vi "Main.vi"() -> ()   [LabVIEW 2021, in "Game of Life.lvlib"]
doc: "This template is for the Queued Message Handler design pattern.\n\nThe Event Handling Loop generates messages based on user interface actions.\n\nThe Message Handling Loop processes messages generated by the Event Handling Loop, or by other messages. The messages are string values, so new messages can be added easily to the Message Cases case structure in the Message Handling Loop. Each message cluster can also provide an optional value for Message Data, which is a variant that can be converted to whatever message-specific data is required."
uses:
  Game of Life.lvlib
  <vilib>/Plug-In SDKs/InstrumentStudio SDK/InstrumentStudioPluginSDK.lvlibp/Plugin Events Enum.ctl
  controls/Data.ctl
  controls/Configuration.ctl
  controls/Game of Life.ctl
  a2cd5499-92a9-455c-b0f9-1db12e3f6067.vi
  aef85ed4-6d5b-4a62-8cd4-232f16e6ae51.vi
  a2cd5499-92a9-455c-b0f9-1db12e3f6067.vi/6651a77e-856e-4bcd-af5a-c0c13b264cc1.vi
  aef85ed4-6d5b-4a62-8cd4-232f16e6ae51.vi/331b549c-fcf8-43d9-8a1e-5b3c0091a99c.vi
  <vilib>/JDP Science/JSONtext/JSON text to Variant.vi
  <vilib>/Utility/error.llb/Error Cluster From Error Code.vi
  <vilib>/JDP Science/JSONtext/Variant to JSON Text.vi
  <vilib>/JDP Science/JSONtext/LVClass Serializer/JSONtext LVClass Serializer.lvclass
  <vilib>/ErrorRing/Error Ring.xnode
  <vilib>/Plug-In SDKs/InstrumentStudio SDK/InstrumentStudioPluginSDK.lvlibp/Plugin Session.lvclass
  <vilib>/Plug-In SDKs/InstrumentStudio SDK/InstrumentStudioPluginSDK.lvlibp
panel:
  in  "Tab Control":enum32{"Game Panel", "Events"}(tab)
  in  "Start":bool
  out "game of life":T1(graph)
  out "generation":u32 caption="Generation"
  in  "update interval":u32=250 caption="Update interval (msec)" min=50
  in  "height":u32=100 caption="Board height" min=10
  in  "width":u32=100 caption="Board width" min=10
  in  "Log Events?":bool
  out "Event Record":i32(listbox)
  in  "Session Id":u64
  # "Enable Logging: Check this box to generate a log file and save the event record."
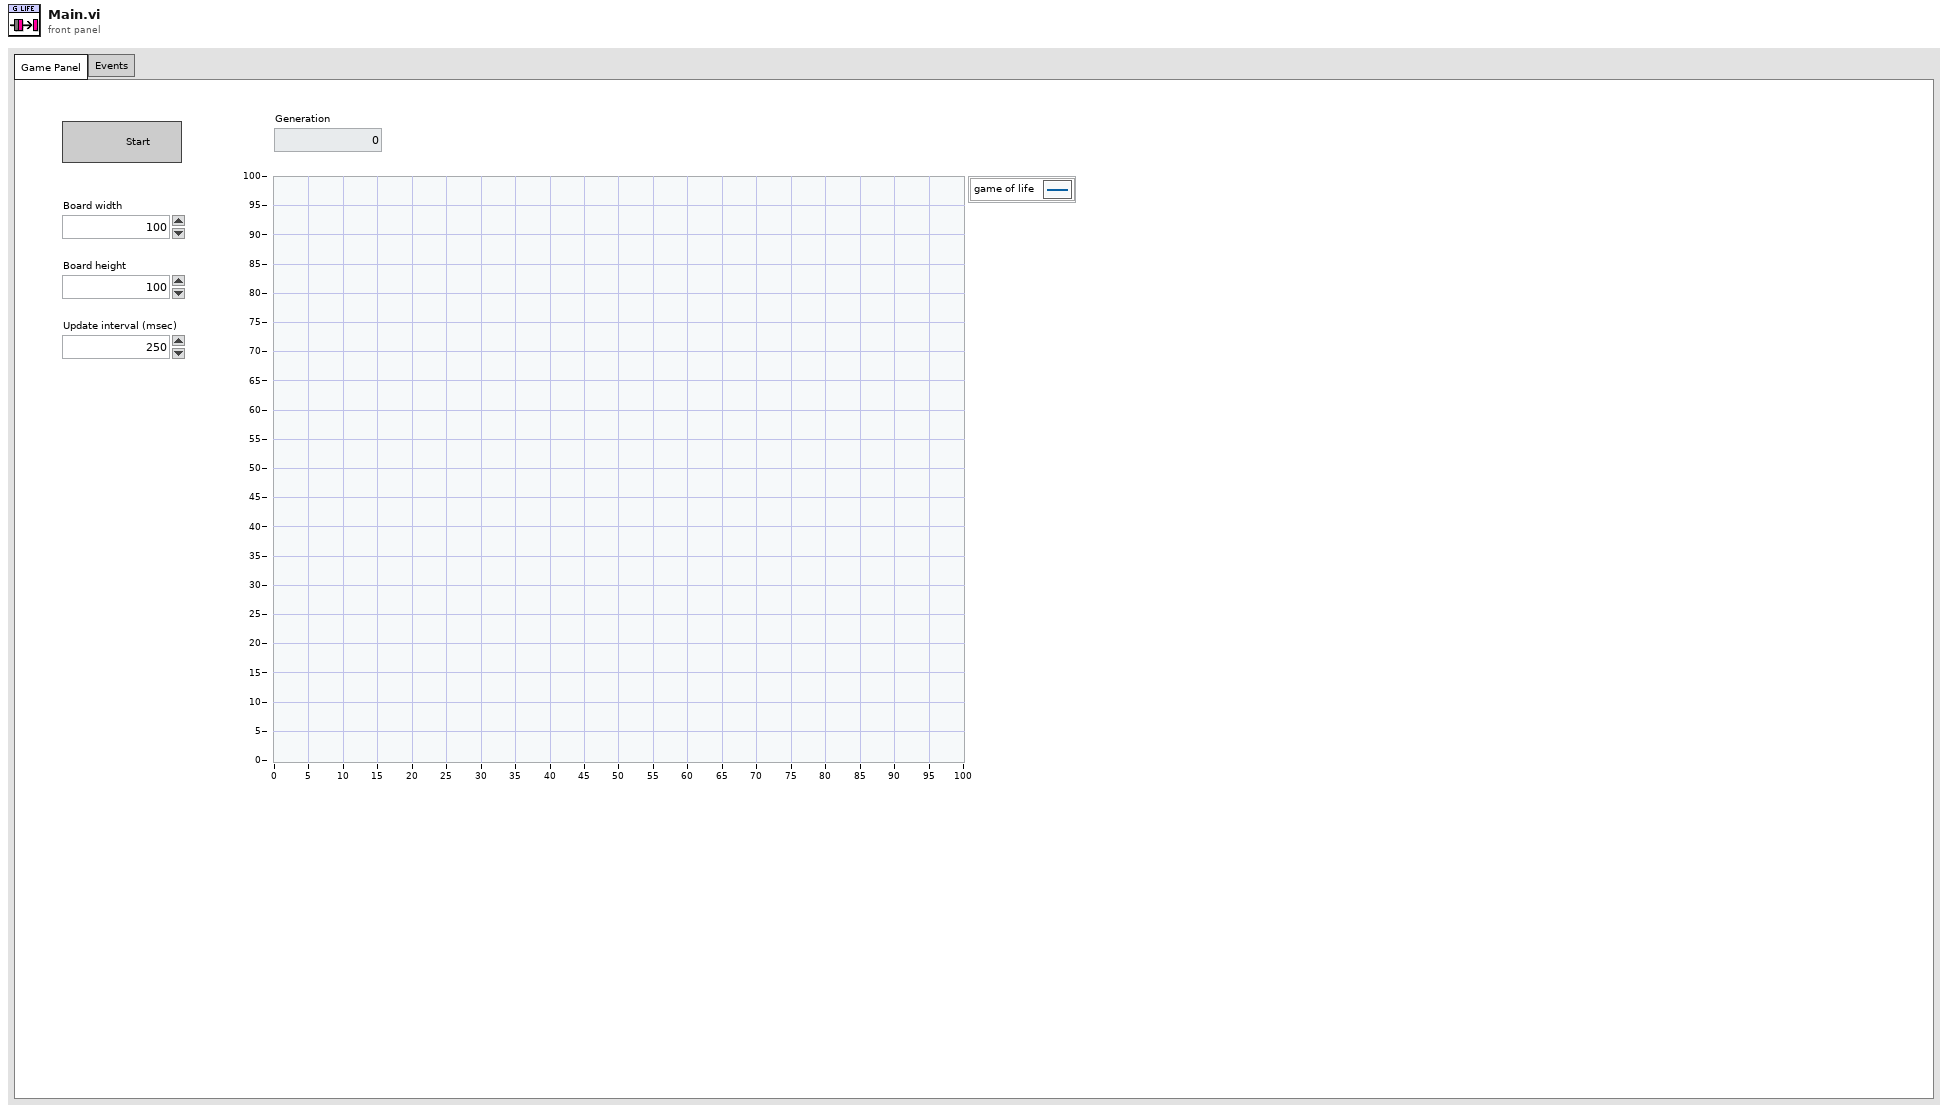
[diagram p1: front panel]
types:
  T1 = typedef "Game of Life.lvlib/Game of Life.ctl" = cluster{"x_data":dbl[], "y_data":dbl[]}
  T2 = typedef "Game of Life.lvlib/Data.ctl" = cluster{"Configuration":T3, "Generation":u32, "Run?":bool, "Cells":bool[][], "Log Events?":bool}
  T3 = typedef "Game of Life.lvlib/Configuration.ctl" = cluster{"Height":u32, "Width":u32, "Update Interval":u32}
  T4 = typedef "InstrumentStudioPluginSDK.lvlibp/Plugin Events Enum.ctl" = enum16{"Shutdown", "Project Saved", "Stop All Outputs"}
  T5 = typedef "InstrumentStudioPluginSDK.lvlibp/Event Registration Refnum.ctl" = refnum<event-registration>
  T6 = typedef "Game of Life.lvlib/All Message Queues.ctl" = cluster{"UI":refnum<queue>}
  T7 = cluster{"Event Refnum":T5, "Event Registration Refnum":refnum<event-registration>}
  T8 = enum8{"Enabled", "Disabled", "Disabled and Grayed Out"}
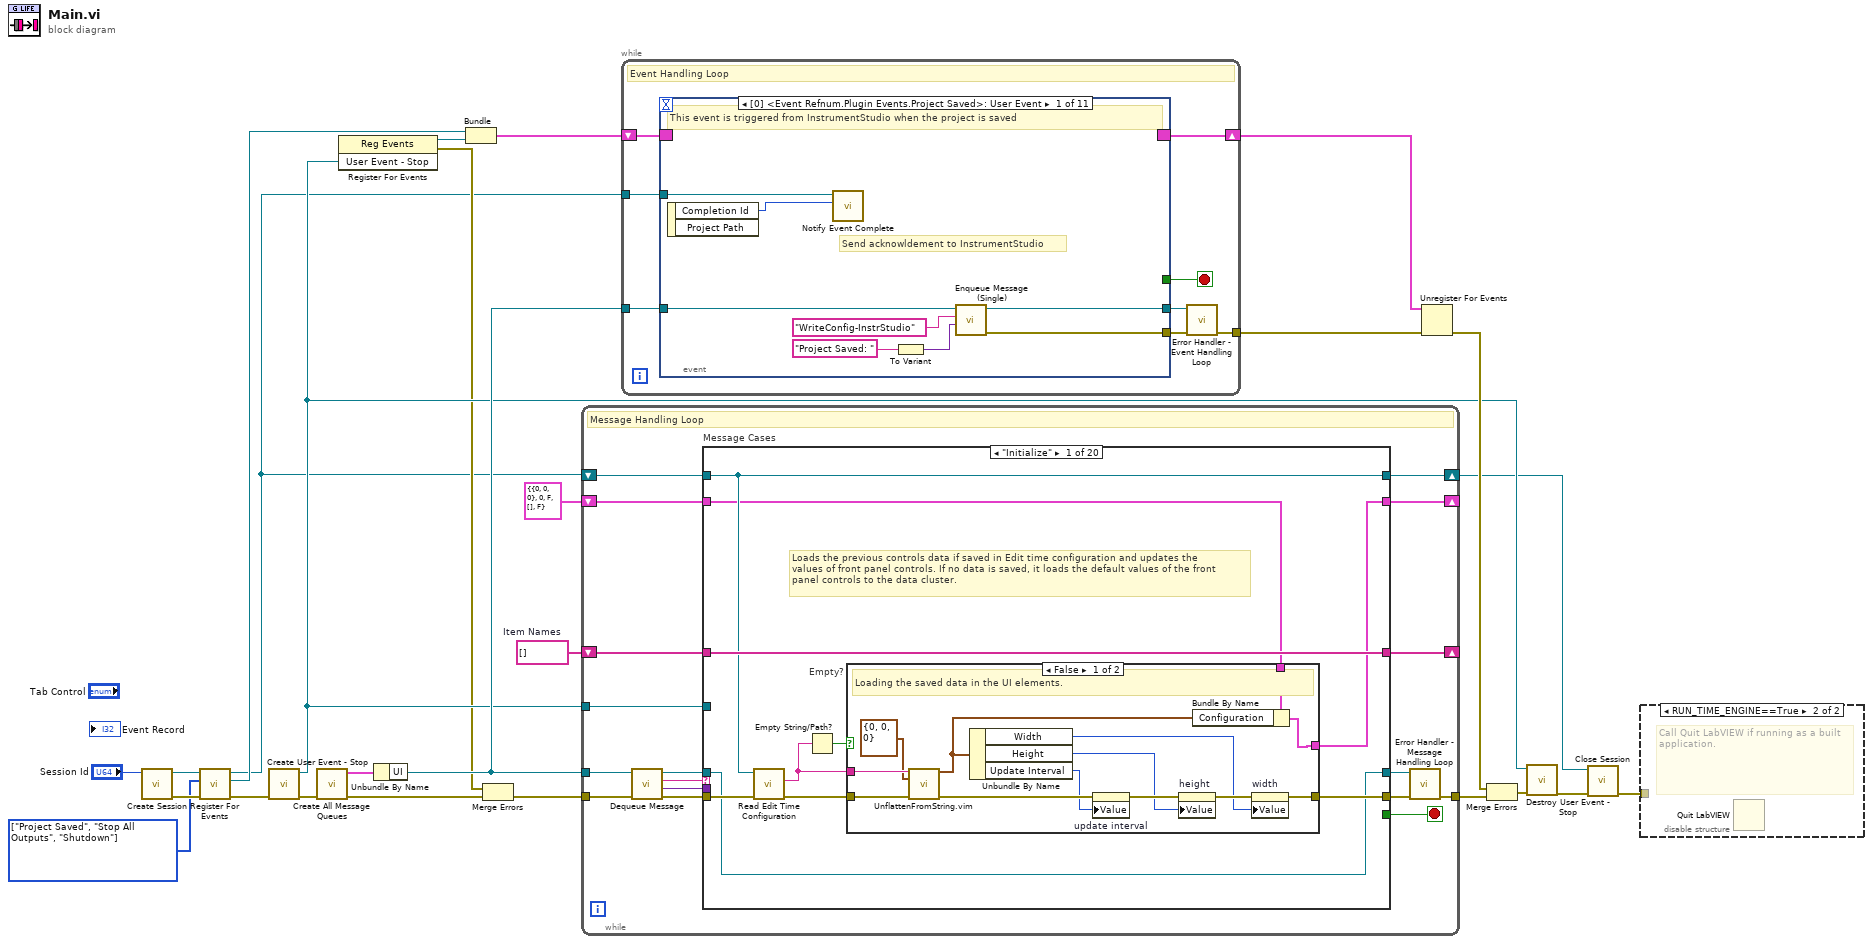
[diagram p0: block diagram]
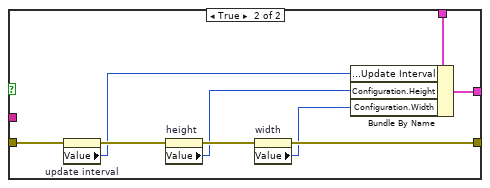
[diagram p3: hidden frame]
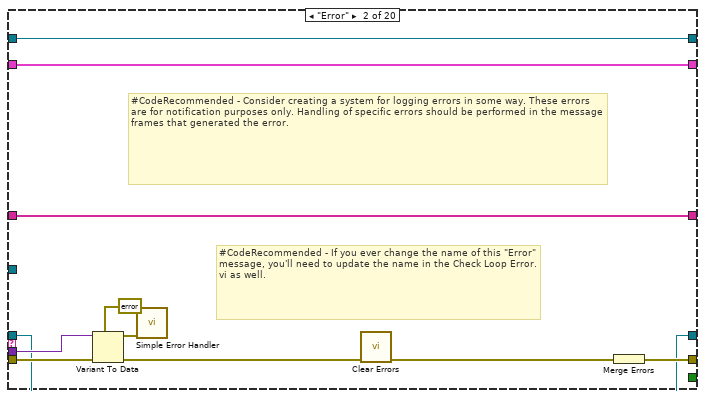
[diagram p4: hidden frame]
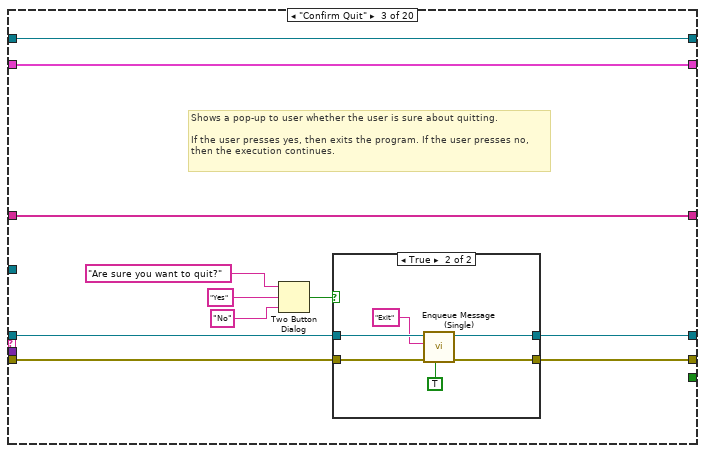
[diagram p5: hidden frame]
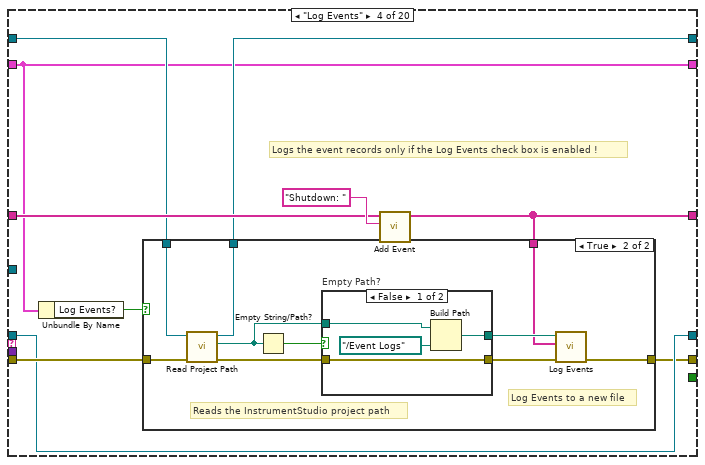
[diagram p7: hidden frame]
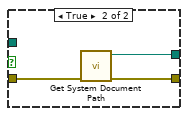
[diagram p9: hidden frame]
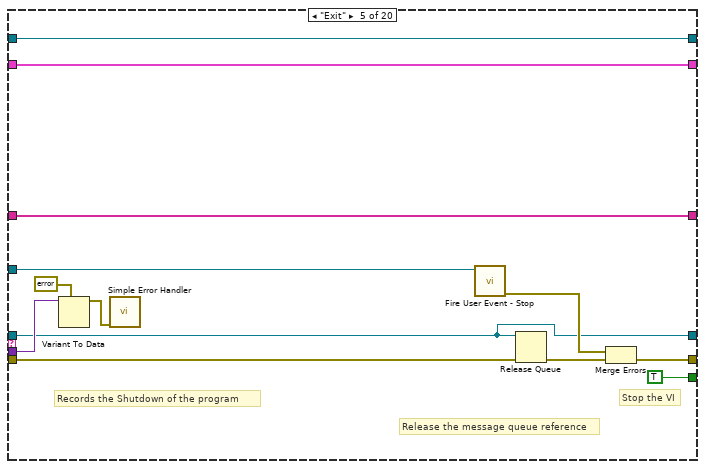
[diagram p10: hidden frame]
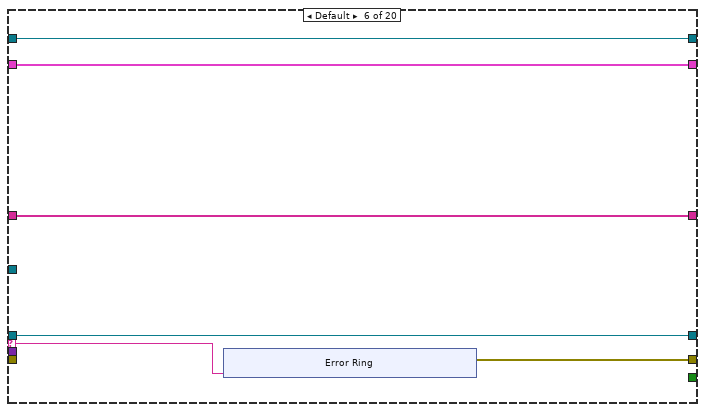
[diagram p11: hidden frame]
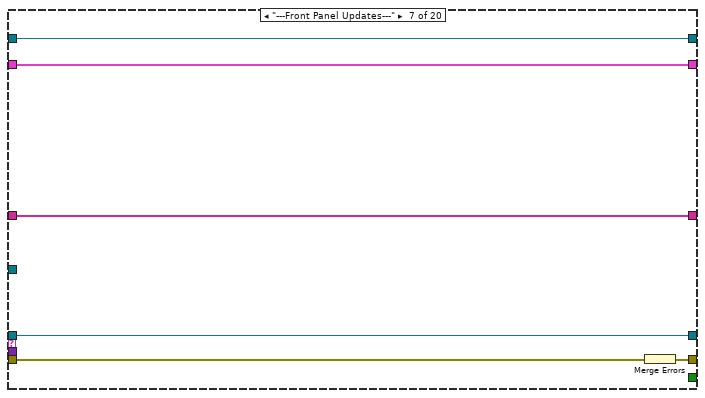
[diagram p12: hidden frame]
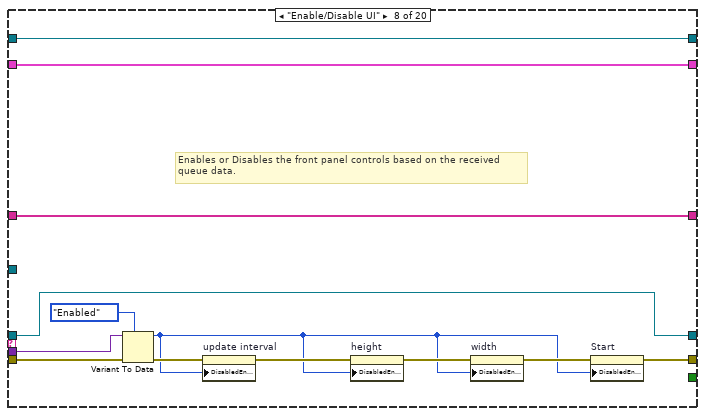
[diagram p13: hidden frame]
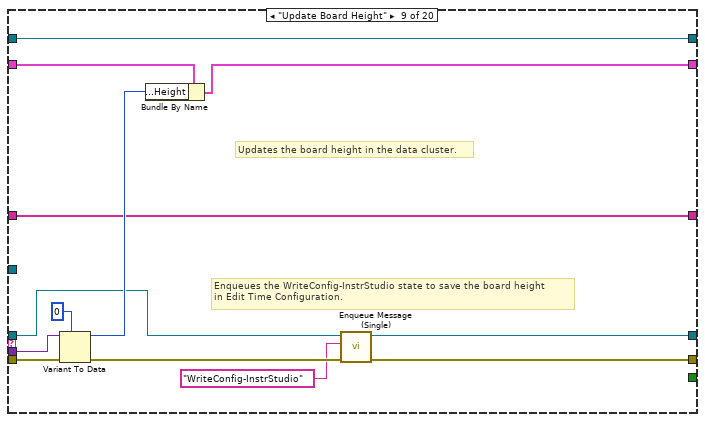
[diagram p14: hidden frame]
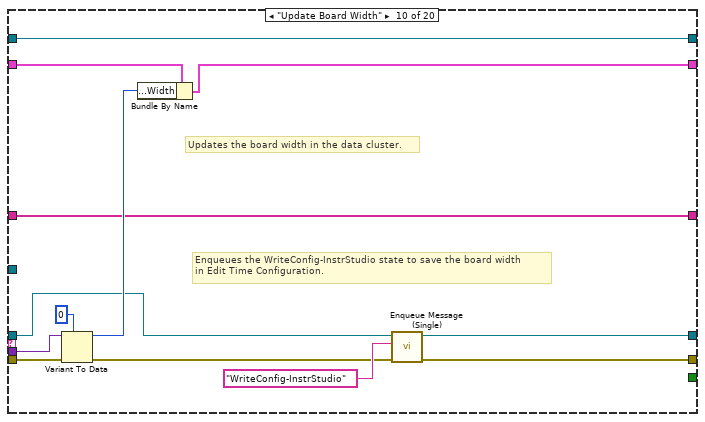
[diagram p15: hidden frame]
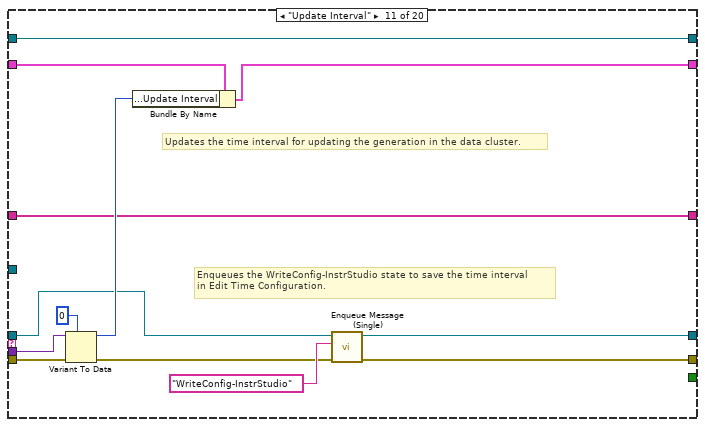
[diagram p16: hidden frame]
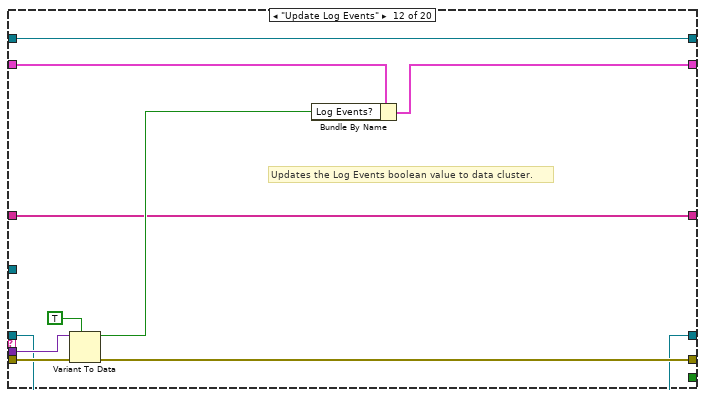
[diagram p17: hidden frame]
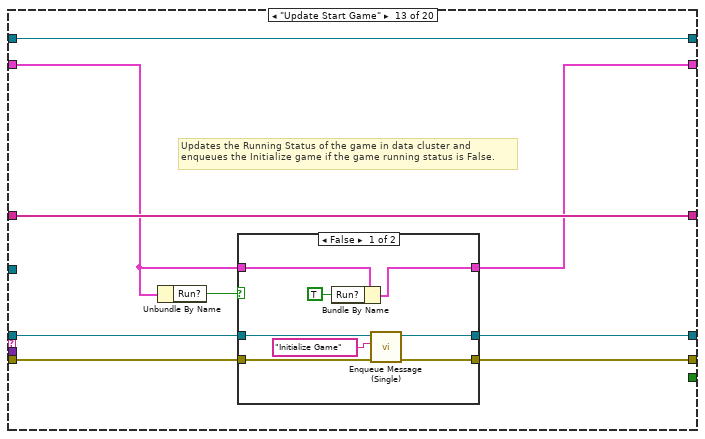
[diagram p18: hidden frame]
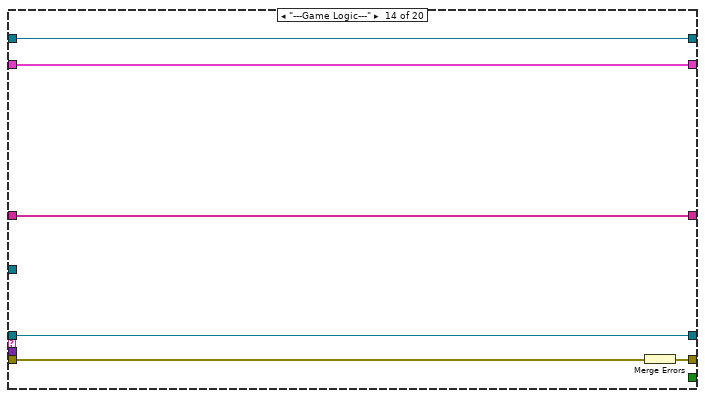
[diagram p20: hidden frame]
diagram:
  w1 = string[] []  # Item Names
  w10 = T4[] [enum."Project Saved", enum."Stop All Outputs", enum."Shutdown"] items=["Shutdown", "Project Saved", "Stop All Outputs"] ("Events To Register")
  n1 = call <vilib>:"Create Session.vi"("Session Id"="Session Id") -> ("error out"=w13:errorcluster, "Session out"=w11:refnum<class "Plugin Session.lvclass">)  [unwired: 6 in, 3 out]
  n2 = call <vilib>:"Register For Events.vi"("error in (no error)"=w13, "Events To Register"=w10, "Session in"=w11) -> ("error out"=w12:errorcluster, "Event Refnum"=w7:T5, "Session out"=w3:refnum<class "Plugin Session.lvclass">)  [unwired: 6 in]
  n3 = call "Create User Event - Stop.vi"("error in (no error)"=w12) -> ("error out"=w22:errorcluster, "User Event - Stop"=w17:refnum<user-event>)  [unwired: 9 in]
  n4 = call "Create All Message Queues.vi"("error in (no error)"=w22) -> ("error out"=w26:errorcluster, "Message Queues out"=w25:T6)  [unwired: 9 in]
  n5 = register-events(w17) -> (reference out=w9:refnum<event-registration>, error out=w15:errorcluster)  [unwired: 2 in]
  n6 = Unbundle By Name(w25) -> ("UI"=w23:refnum<queue>)
  n7 = Bundle("Event Refnum"=w7, "Event Registration Refnum"=w9) -> (w8:T7)  [unwired: 1 in]
  n8 = Merge Errors(w15, w26) -> (w16:errorcluster)
  n9 = while {
    tunnel: w23 -> [w37]
    tunnel: w17 -> [w42]
    tunnel: w16 -> [w41]
    tunnel: [w35] -> w24
    shift-right: [w32] -> w6
    shift-left: w3 -> [w33]
    shift-right: [w31] -> _
    shift-left: T2 {"Configuration"={"Height"=0, "Width"=0, "Update Interval"=0}, "Generation"=0, "Run?"=FALSE, "Cells"=[], "Log Events?"=FALSE} ("Configuration") -> [w30]
    shift-right: [w28] -> _
    shift-left: w1 -> [w29]
    stop <- w43 stop-if-true
    # "Message Handling Loop"
    n10 = call "Dequeue Message.vi"("error in (no error)"=w41, "Message Queue"=w37) -> ("error out"=w40:errorcluster, "Message Data"=w38:variant, "Message"=w39:string, "dup Message Queue"=w36:refnum<queue>)  [unwired: 6 in]
    n11 = case "Message Cases" shown="\"Initialize\"" w39 {
      selector: w39 -> [_ _ _ _ _ w151 _ _ _ _ _ _ _ _ _ _ _ _ _ _]
      tunnel: w36 -> [w46 w76 w95 w110 w136 w147 w160 w167 w180 w193 w205 w222 w229 w248 w267 w280 w314 w330 w339 w351]
      tunnel: w40 -> [w49 w86 w97 w113 w135 _ w165 w171 w190 w203 w216 w225 w235 w253 w265 w285 w319 w332 w341 w350]
      tunnel: [w53 w81 w96 w109 w144 w152 w164 w173 w182 w192 w207 w226 w230 w252 w268 w281 w318 w328 w342 w357] -> w34
      tunnel: [_ _ _ _ TRUE _ _ _ _ _ _ _ _ _ _ _ _ _ _ _] -> w43
      tunnel: w38 -> [_ w85 _ _ w139 _ _ w170 w189 w202 w215 w224 _ _ _ _ _ _ _ w348]
      tunnel: w42 -> [_ _ _ _ w143 _ _ _ _ _ _ _ _ _ _ _ _ _ _ _]
      tunnel: w33 -> [w47 w80 w94 w111 w138 w150 w163 w178 w191 w204 w217 w227 w236 w251 w273 w286 w317 w336 w344 w359]
      tunnel: [w47 w80 w94 w112 w138 w150 w163 w178 w191 w204 w217 w227 w236 w251 w273 w286 w317 w336 w343 w358] -> w32
      tunnel: [w45 w79 w93 w107 w137 w149 w162 w177 w186 w200 w213 w221 w231 w250 w272 w274 w316 w334 w338 w352] -> w31
      tunnel: w30 -> [w44 w79 w93 w107 w137 w149 w162 w177 w185 w199 w212 w220 w232 w250 w271 w278 w316 w333 w338 w352]
      tunnel: w29 -> [w48 w77 w92 w114 w134 w148 w161 w166 w184 w197 w210 w218 w234 w249 w270 w284 w315 w324 w340 w349]
      tunnel: [w48 w77 w92 w108 w134 w148 w161 w166 w184 w197 w210 w218 w234 w249 w270 w284 w315 w325 w340 w353] -> w28
      tunnel: [w46 w76 w91 w110 w136 w147 w160 w167 w181 w194 w206 w222 w228 w248 w266 w277 w314 w326 w339 w351] -> w27
      frame "Initialize" {
        # "Loads the previous controls data if saved in Edit time configuration and updates the\nvalues of front panel controls. If no data is saved, it loads the default values of the front\npanel controls to the data cluster."
        # "Initialize - All initialization work should take place in this message, since other loops can potentially enqueue messages that execute immediately after this one."
        n12 = call <vilib>:"Read Edit Time Configuration.vi"("error in (no error)"=w49, "Session in"=w47) -> ("error out"=w50:errorcluster, "Edit Time Configuration"=w51:string)  [unwired: 7 in, 1 out]
        n13 = Empty String/Path?(string/path=w51) -> (empty?=w52:bool)
        n14 = case "Empty?" shown="False" w52 {
          tunnel: [w59 w72] -> w53
          tunnel: w50 -> [w65 w71]
          tunnel: w51 -> [w66 _]
          tunnel: w44 -> [w56 w75]
          tunnel: [w55 w69] -> w45
          frame False {
            # "Loading the saved data in the UI elements."
            n15 = call "UnflattenFromString.vim"("Flattened Data"=w66, "Data Type"=T3 {"Height"=0, "Width"=0, "Update Interval"=0} ("Configuration"), "error in"=w65) -> ("Data Out"=w54:T3, "error out"=w64:errorcluster)  [unwired: 11 in]
            n16 = Unbundle By Name(w54) -> ("Width"=w58:u32, "Height"=w61:u32, "Update Interval"=w63:u32)
            n17 = property on="update interval" class="DigNum (strict)"(error in=w64, "Value"=w63) -> (error out=w62:errorcluster)  [unwired: 1 in, 1 out]
            n18 = property on="height" class="DigNum (strict)"(error in=w62, "Value"=w61) -> (error out=w60:errorcluster)  [unwired: 1 in, 1 out]
            n19 = Bundle By Name(cluster=w56, "Configuration"=w54) -> (w55:T2)
            n20 = property on="width" class="DigNum (strict)"(error in=w60, "Value"=w58) -> (error out=w59:errorcluster)  [unwired: 1 in, 1 out]
          }
          frame True {
            n21 = property on="update interval" class="DigNum (strict)"(error in=w71) -> (error out=w74:errorcluster, "Value"=w70:u32)  [unwired: 1 in, 1 out]
            n22 = property on="height" class="DigNum (strict)"(error in=w74) -> (error out=w73:errorcluster, "Value"=w68:u32)  [unwired: 1 in, 1 out]
            n23 = property on="width" class="DigNum (strict)"(error in=w73) -> (error out=w72:errorcluster, "Value"=w67:u32)  [unwired: 1 in, 1 out]
            n24 = Bundle By Name(cluster=w75, "Configuration.Update Interval"=w70, "Configuration.Height"=w68, "Configuration.Width"=w67) -> (w69:T2)
          }
        }
      }
      frame "Error" {
        # "#CodeRecommended - If you ever change the name of this \"Error\" message, you'll need to update the name in the Check Loop Error.vi as well."
        # "#CodeRecommended - Consider creating a system for logging errors in some way. These errors are for notification purposes only. Handling of specific errors should be performed in the message frames that generated the error."
        # "Error - Display an error dialog. This message is sent by the \"Error Handler\" VIs at the end of other loops in this application."
        n25 = Variant To Data(error in=w86, type=errorcluster {"status"=FALSE, "code"=0, "source"=""} ("error constant"), Variant=w85) -> (data=w83:errorcluster, error out=w82:errorcluster)
        n26 = call <vilib>:"Simple Error Handler.vi"("error in (no error)"=w83) -> ()  [unwired: 4 in, 5 out]
        n27 = call <vilib>:"Clear Errors.vi"("error in (no error)"=w82) -> ("error out"=w78:errorcluster)  [unwired: 5 in, 1 out]
        n28 = Merge Errors(w78) -> (w81:errorcluster)
      }
      frame "Confirm Quit" {
        # "Shows a pop-up to user whether the user is sure about quitting. \n\nIf the user presses yes, then exits the program. If the user presses no,\nthen the execution continues."
        # "Confirm Quit - Message that can confirm whether or not the user wants to exit the application."
        n29 = Two Button Dialog(message="Are sure you want to quit?", 1:"No" ("F button name (\"Cancel\")"), 2:"Yes" ("T button name (\"OK\")")) -> (T button?=w87:bool)
        n30 = case shown="True" w87 {
          tunnel: w97 -> [w98 w105]
          tunnel: [w98 w104] -> w96
          tunnel: w95 -> [w99 w103]
          tunnel: [w99 w100] -> w91
          frame False {
          }
          frame True {
            n31 = call "Enqueue Message (Single).vi"("Priority Message? (F)"=TRUE, "error in (no error)"=w105, "Message"="Exit", "Message Queue"=w103) -> ("error out"=w104:errorcluster, "dup Message Queue"=w100:refnum<queue>)  [unwired: 6 in]
          }
        }
      }
      frame "Log Events" {
        # "Logs the event records only if the Log Events check box is enabled !"
        n32 = Unbundle By Name(w107) -> ("Log Events?"=w106:bool)
        n33 = call "Add Event.vi"("Event Tag"="Shutdown: ", "Item Names in"=w114) -> ("Item Names out"=w108:string[])  [unwired: 9 in]
        n34 = case shown="True" w106 {
          tunnel: w113 -> [w117 w127]
          tunnel: [w116 w126] -> w112
          tunnel: w111 -> [w116 w125]
          tunnel: [w117 w120] -> w109
          tunnel: w108 -> [_ w118]
          frame False {
          }
          frame True {
            # "Log Events to a new file"
            # "Reads the InstrumentStudio project path"
            n35 = call <vilib>:"Read Project Path.vi"("error in (no error)"=w127, "Session in"=w125) -> ("error out"=w123:errorcluster, "Project Path"=w122:path, "Session out"=w126:refnum<class "Plugin Session.lvclass">)  [unwired: 7 in]
            n36 = Empty String/Path?(string/path=w122) -> (empty?=w124:bool)
            n37 = case "Empty Path?" shown="False" w124 {
              tunnel: w123 -> [w131 w132]
              tunnel: w122 -> [w130 _]
              tunnel: [w128 w133] -> w121
              tunnel: [w131 w132] -> w119
              frame False {
                n38 = Build Path(base path=w130, name or relative path=path "../Event Logs") -> (appended path=w128:path)
              }
              frame True {
                n39 = call "Get System Document Path.vi"() -> ("Public Path"=w133:path)  [unwired: 11 in]
              }
            }
            n40 = call "Log Events.vi"("error in"=w119, "Item Names"=w118, "Event Folder Path"=w121) -> ("error out"=w120:errorcluster)  [unwired: 8 in]
          }
        }
      }
      frame "Exit" {
        # "Records the Shutdown of the program"
        # "Stop the VI"
        # "Release the message queue reference"
        # "Exit - Exit the application."
        n41 = Variant To Data(type=errorcluster {"status"=FALSE, "code"=0, "source"=""} ("error constant"), Variant=w139) -> (data=w140:errorcluster)  [unwired: 1 in, 1 out]
        n42 = call <vilib>:"Simple Error Handler.vi"("error in (no error)"=w140) -> ()  [unwired: 4 in, 5 out]
        n43 = call "Fire User Event - Stop.vi"("User Event - Stop"=w143) -> ("error out"=w142:errorcluster)  [unwired: 10 in]
        n44 = Release Queue(queue=w136, error in (no error)=w135) -> (error out=w145:errorcluster)  [unwired: 1 in, 2 out]
        n45 = Merge Errors(w142, w145) -> (w144:errorcluster)
      }
      frame Default {
        # "'Default' case only runs if there is a message that isn't defined in any of the other cases.  Output a programming error."
        n46 = xnode "Error Ring"("parameter 0"=w151) -> ("error out"=w152:errorcluster)
      }
      frame "---Front Panel Updates---" {
        # "Duplicate this frame when creating new messages.  Change this comment in the duplicated frame to describe this message."
        n47 = Merge Errors(w165) -> (w164:errorcluster)
      }
      frame "Enable/Disable UI" {
        # "Enables or Disables the front panel controls based on the received \nqueue data."
        n48 = Variant To Data(error in=w171, type=T8."Enabled" ("Disabled"), Variant=w170) -> (data=w168:T8, error out=w172:errorcluster)
        n49 = property on="update interval" class="DigNum (strict)"(error in=w172, "DisabledEnum"=w168) -> (error out=w176:errorcluster)  [unwired: 1 in, 1 out]
        n50 = property on="height" class="DigNum (strict)"(error in=w176, "DisabledEnum"=w168) -> (error out=w175:errorcluster)  [unwired: 1 in, 1 out]
        n51 = property on="width" class="DigNum (strict)"(error in=w175, "DisabledEnum"=w168) -> (error out=w174:errorcluster)  [unwired: 1 in, 1 out]
        n52 = property on="Start" class="Bool"(error in=w174, "DisabledEnum"=w168) -> (error out=w173:errorcluster)  [unwired: 1 in, 1 out]
      }
      frame "Update Board Height" {
        # "Enqueues the WriteConfig-InstrStudio state to save the board height\nin Edit Time Configuration."
        # "Updates the board height in the data cluster."
        n53 = Variant To Data(error in=w190, type=u32 0 ("wid"), Variant=w189) -> (data=w187:u32, error out=w183:errorcluster)
        n54 = Bundle By Name(cluster=w185, "Configuration.Height"=w187) -> (w186:T2)
        n55 = call "Enqueue Message (Single).vi"("error in (no error)"=w183, "Message"="WriteConfig-InstrStudio", "Message Queue"=w180) -> ("error out"=w182:errorcluster, "dup Message Queue"=w181:refnum<queue>)  [unwired: 7 in]
      }
      frame "Update Board Width" {
        # "Enqueues the WriteConfig-InstrStudio state to save the board width\nin Edit Time Configuration."
        # "Updates the board width in the data cluster."
        n56 = Variant To Data(error in=w203, type=u32 0 ("wid"), Variant=w202) -> (data=w198:u32, error out=w195:errorcluster)
        n57 = Bundle By Name(cluster=w199, "Configuration.Width"=w198) -> (w200:T2)
        n58 = call "Enqueue Message (Single).vi"("error in (no error)"=w195, "Message"="WriteConfig-InstrStudio", "Message Queue"=w193) -> ("error out"=w192:errorcluster, "dup Message Queue"=w194:refnum<queue>)  [unwired: 7 in]
      }
      frame "Update Interval" {
        # "Enqueues the WriteConfig-InstrStudio state to save the time interval\nin Edit Time Configuration."
        # "Updates the time interval for updating the generation in the data cluster."
        n59 = Variant To Data(error in=w216, type=u32 0 ("wid"), Variant=w215) -> (data=w211:u32, error out=w208:errorcluster)
        n60 = Bundle By Name(cluster=w212, "Configuration.Update Interval"=w211) -> (w213:T2)
        n61 = call "Enqueue Message (Single).vi"("error in (no error)"=w208, "Message"="WriteConfig-InstrStudio", "Message Queue"=w205) -> ("error out"=w207:errorcluster, "dup Message Queue"=w206:refnum<queue>)  [unwired: 7 in]
      }
      frame "Update Log Events" {
        # "Updates the Log Events boolean value to data cluster."
        n62 = Variant To Data(error in=w225, type=TRUE, Variant=w224) -> (data=w219:bool, error out=w226:errorcluster)
        n63 = Bundle By Name(cluster=w220, "Log Events?"=w219) -> (w221:T2)
      }
      frame "Update Start Game" {
        # "Updates the Running Status of the game in data cluster and\nenqueues the Initialize game if the game running status is False."
        n64 = Unbundle By Name(w232) -> ("Run?"=w233:bool)
        n65 = case shown="False" w233 {
          tunnel: w235 -> [w239 w246]
          tunnel: w232 -> [w244 w247]
          tunnel: [w243 w247] -> w231
          tunnel: [w240 w246] -> w230
          tunnel: w229 -> [w241 w245]
          tunnel: [w238 w245] -> w228
          frame False {
            n66 = Bundle By Name(cluster=w244, "Run?"=TRUE) -> (w243:T2)
            n67 = call "Enqueue Message (Single).vi"("error in (no error)"=w239, "Message"="Initialize Game", "Message Queue"=w241) -> ("error out"=w240:errorcluster, "dup Message Queue"=w238:refnum<queue>)  [unwired: 7 in]
          }
          frame True {
          }
        }
      }
      frame "---Game Logic---" {
        # "Duplicate this frame when creating new messages.  Change this comment in the duplicated frame to describe this message."
        n68 = Merge Errors(w253) -> (w252:errorcluster)
      }
      frame "Initialize Game" {
        w264 = -1.0 ("X Scale.Range:Minimum")
        # "Generate an initial random \nliving cells in a 2D array"
        # "Initializes the Board"
        n69 = Unbundle By Name(w271) -> ("Configuration.Width"=w262:u32, "Configuration.Height"=w260:u32)
        n70 = To Double Precision Float(number=w262) -> (double precision float=w263:dbl)
        n71 = To Double Precision Float(number=w260) -> (double precision float=w261:dbl)
        n72 = call "Initialize Game.vi"("Height"=w260, "Width"=w262) -> ("Array"=w269:bool[][])  [unwired: 9 in]
        n73 = property on="game of life" class="XYGraph (strict)"(error in=w265, "XScale.Minimum"=w264, "XScale.Maximum"=w263, "YScale.Minimum"=w264, "YScale.Maximum"=w261, "Value"=T1 {"x_data"=[], "y_data"=[]} ("game of life")) -> (error out=w259:errorcluster)  [unwired: 1 in, 1 out]
        n74 = Bundle By Name(cluster=w271, "Generation"=u32 0, "Cells"=w269) -> (w272:T2)
        n75 = call "Enum to Variant Array.vi"("Disabled"=T8."Disabled and Grayed Out") -> ("Message Data Array"=w254:variant[])  [unwired: 10 in]
        n76 = call "Enqueue Message (Array).vi"("error in (no error)"=w259, "Message Data Array"=w254, "Message Array"=string[] ["Enable/Disable UI", "UpdateRunningFlag-InstrStudio", "Game of Life"], "Message Queue"=w267) -> ("error out"=w268:errorcluster, "dup Message Queue"=w266:refnum<queue>)  [unwired: 6 in]
      }
      frame "Game of Life" {
        # "If the stop condition is met, then stops execution of the \ngame logic. If not, keeps executing the game logic by \nenqueueing the present state."
        # "Generates the next generation of living cells by\nappliying game logic to the current generation \nliving cells with the specified time interval."
        n77 = in-place {
          in-place-border: w285 -> [w295]
          in-place-border: [w291] -> w282
          in-place-border: [w290] -> w283
          in-place-border: [w289] -> w279
          in-place-border: [w287] -> w276
          n78 = in-place-cluster #1(w278) -> ("Cells"=w294:bool[][], "Generation"=w293:u32, "Configuration.Update Interval"=w288:u32)
          n79 = call "Wrap Next Generation.vi"("error in"=w295, "Update Interval"=w288, "generation in"=w293, "cells in"=w294) -> ("error out"=w291:errorcluster, "game of life"=w289:T1, "generation out"=w287:u32, "cells out"=w292:bool[][], "Stop?"=w290:bool)  [unwired: 3 in]
          n80 = in-place-cluster #1("Cells"=w292, "Generation"=w287, "Configuration.Update Interval"=w288) -> (w275:T2)
        }
        n81 = case "Stop?" shown="False" w283 {
          tunnel: w282 -> [w300 w309]
          tunnel: [w303 w310] -> w281
          tunnel: w280 -> [w302 w308]
          tunnel: w279 -> [w297 _]
          tunnel: [w299 w307] -> w277
          tunnel: w276 -> [w298 _]
          tunnel: w275 -> [w296 w305]
          tunnel: [w296 w306] -> w274
          frame False {
            n82 = call "Enqueue Message (Single).vi"("error in (no error)"=w300, "Message"="Game of Life", "Message Queue"=w302) -> ("error out"=w303:errorcluster, "dup Message Queue"=w299:refnum<queue>)  [unwired: 7 in]
            "generation" <- w298
            "game of life" <- w297
          }
          frame True {
            n83 = call "Enum to Variant Array.vi"("Disabled"=T8."Enabled") -> ("Message Data Array"=w313:variant[])  [unwired: 10 in]
            n84 = Bundle By Name(cluster=w305, "Run?"=FALSE) -> (w306:T2)
            n85 = call "Enqueue Message (Array).vi"("error in (no error)"=w309, "Message Data Array"=w313, "Message Array"=string[] ["Enable/Disable UI", "UpdateRunningFlag-InstrStudio"], "Message Queue"=w308) -> ("error out"=w310:errorcluster, "dup Message Queue"=w307:refnum<queue>)  [unwired: 6 in]
          }
        }
      }
      frame "---Instrument Studio Interaction---" {
        # "Duplicate this frame when creating new messages.  Change this comment in the duplicated frame to describe this message."
        n86 = Merge Errors(w319) -> (w318:errorcluster)
      }
      frame "StopAllOutputs" {
        # "Flush the Queue to stop game logic execution"
        # "Updates the Running Status of the game in data cluster"
        # "Updates the Event Record indicator with current event."
        n87 = call "Add Event.vi"("Event Tag"="Stop All Outputs: ", "Item Names in"=w324) -> ("Item Names out"=w325:string[])  [unwired: 9 in]
        n88 = property on="Event Record" class="LstBox (strict)"(error in=w332, "Item Names"=w325) -> (error out=w331:errorcluster)  [unwired: 1 in, 1 out]
        n89 = Bundle By Name(cluster=w333, "Run?"=FALSE) -> (w334:T2)
        n90 = Flush Queue(queue=w330, error in (no error)=w331) -> (queue out=w327:refnum<queue>, error out=w329:errorcluster)  [unwired: 1 out]
        n91 = call "Enum to Variant Array.vi"("Disabled"=T8."Enabled") -> ("Message Data Array"=w321:variant[])  [unwired: 10 in]
        n92 = call "Enqueue Message (Array).vi"("error in (no error)"=w329, "Message Data Array"=w321, "Message Array"=string[] ["Enable/Disable UI", "UpdateRunningFlag-InstrStudio"], "Message Queue"=w327) -> ("error out"=w328:errorcluster, "dup Message Queue"=w326:refnum<queue>)  [unwired: 6 in]
      }
      frame "UpdateRunningFlag-InstrStudio" {
        # "Updates the running flag in \nInstrumentStudio"
        n93 = Unbundle By Name(w338) -> ("Run?"=w337:bool)
        n94 = call <vilib>:"Update Running State.vi"("error in (no error)"=w341, "Is Running"=w337, "Plugin Session in"=w344) -> ("error out"=w342:errorcluster, "Plugin Session out"=w343:refnum<class "Plugin Session.lvclass">)  [unwired: 7 in]
      }
      frame "WriteConfig-InstrStudio" {
        # "Saving the control inputs\nin the instrumentStudio object"
        n95 = Equal?(x=w348, y=variant) -> (x = y?=w346:bool)
        n96 = case "Empty Variant?" shown="False" w346 {
          tunnel: [w367 w368] -> w354
          tunnel: [w366 w369] -> w353
          tunnel: w350 -> [w362 w368]
          tunnel: w348 -> [w361 _]
          tunnel: w349 -> [w365 w369]
          frame False {
            # "Records the project save event in event record indicator."
            n97 = Variant To Data(error in=w362, type="", Variant=w361) -> (data=w360:string, error out=w363:errorcluster)
            n98 = call "Add Event.vi"("Event Tag"=w360, "Item Names in"=w365) -> ("Item Names out"=w366:string[])  [unwired: 9 in]
            n99 = property on="Event Record" class="LstBox (strict)"(error in=w363, "Item Names"=w366) -> (error out=w367:errorcluster)  [unwired: 1 in, 1 out]
          }
          frame True {
          }
        }
        n100 = Unbundle By Name(w352) -> ("Configuration"=w345:T3)
        n101 = call "FlattenToString.vim"("Anything"=w345, "error in"=w354) -> ("Flattened Data"=w356:string, "error out"=w355:errorcluster)  [unwired: 12 in]
        n102 = call <vilib>:"Write Edit Time Configuration.vi"("error in (no error)"=w355, "Edit Time Configuration"=w356, "Session in"=w359) -> ("error out"=w357:errorcluster, "Session out"=w358:refnum<class "Plugin Session.lvclass">)  [unwired: 7 in]
      }
    }
    n103 = call "Error Handler - Message Handling Loop.vi"("error in (no error)"=w34, "Message Queue"=w27) -> ("dup error in"=w35:errorcluster)  [unwired: 8 in, 1 out]
  }
  n104 = while {
    tunnel: w23 -> [w377]
    shift-right: [w375] -> w19
    shift-left: w8 -> [w376]
    tunnel: [w371] -> w18
    tunnel: w3 -> [w370]
    stop <- w373 stop-if-true
    # "Event Handling Loop"
    n105 = event shown="[0] <Event Refnum.Plugin Events.Project Saved>: User Event" {
      selector: w376 -> [_ _ _ _ _ _ _ _ _ _ _]
      dyn-events: [_ _ _ _ _ _ _ _ _ _ _] -> w375
      timeout: _ -> [_ _ _ _ _ _ _ _ _ _ _]
      tunnel: [_ _ _ _ _ _ _ _ _ _ TRUE ("Discard?")] -> w373
      tunnel: w377 -> [w382 w390 w395 w401 w407 w413 w418 w422 w429 w431 w433]
      tunnel: [w380 w387 w396 w400 w406 w412 _ w421 w428 _ _] -> w374
      tunnel: [w381 w388 w397 w402 w408 w414 w417 w423 w427 w431 w433] -> w372
      tunnel: w370 -> [w385 w392 _ _ _ _ _ _ _ _ _]
      event User Event {
        # "Send acknowldement to InstrumentStudio"
        # "This event is triggered from InstrumentStudio when the project is saved"
        n106 = event-data() -> ("Completion Id"=w384:i64)  [unwired: 1 in, 1 out]
        n107 = call <vilib>:"Notify Event Complete.vi"("Completion Id"=w384, "Session in"=w385) -> ()  [unwired: 8 in, 2 out]
        n108 = To Variant(anything="Project Saved: " ("string")) -> (Variant=w379:variant)
        n109 = call "Enqueue Message (Single).vi"("Message Data"=w379, "Message"="WriteConfig-InstrStudio", "Message Queue"=w382) -> ("error out"=w380:errorcluster, "dup Message Queue"=w381:refnum<queue>)  [unwired: 7 in]
      }
      event User Event {
        # "Send acknowldement to InstrumentStudio"
        # "This event is triggered from InstrumentStudio when the project Stop All Outputs button is pressed"
        n110 = event-data() -> ("Completion Id"=w391:i64)  [unwired: 1 in]
        n111 = call <vilib>:"Notify Event Complete.vi"("Completion Id"=w391, "Session in"=w392) -> ()  [unwired: 8 in, 2 out]
        n112 = call "Enqueue Message (Single).vi"("Priority Message? (F)"=TRUE, "Message"="StopAllOutputs", "Message Queue"=w390) -> ("error out"=w387:errorcluster, "dup Message Queue"=w388:refnum<queue>)  [unwired: 7 in]
      }
      event User Event {
        # "This event doesn't need acknowledgement from plugin"
        # "This event is triggered when softpanel/instrumentstudio is closed"
        n113 = event-data() -> ()  [unwired: 1 in, 1 out]
        n114 = call "Enqueue Message (Array).vi"("Priority Message? Array"=bool[] [TRUE, TRUE], "Message Array"=string[] ["Log Events", "Exit"], "Message Queue"=w395) -> ("error out"=w396:errorcluster, "dup Message Queue"=w397:refnum<queue>)  [unwired: 7 in]
      }
      event "height": Value Change {
        # "Captures value change in height and sends data to Message Handling Loop"
        n115 = event-data() -> ("NewVal"=w399:u32)  [unwired: 1 in]
        n116 = To Variant(anything=w399) -> (Variant=w398:variant)
        n117 = call "Enqueue Message (Single).vi"("Message Data"=w398, "Message"="Update Board Height", "Message Queue"=w401) -> ("error out"=w400:errorcluster, "dup Message Queue"=w402:refnum<queue>)  [unwired: 7 in]
      }
      event "width": Value Change {
        # "Captures value change in width and sends data to Message Handling Loop"
        n118 = event-data() -> ("NewVal"=w405:u32)  [unwired: 1 in]
        n119 = To Variant(anything=w405) -> (Variant=w404:variant)
        n120 = call "Enqueue Message (Single).vi"("Message Data"=w404, "Message"="Update Board Width", "Message Queue"=w407) -> ("error out"=w406:errorcluster, "dup Message Queue"=w408:refnum<queue>)  [unwired: 7 in]
      }
      event "update interval": Value Change {
        # "Captures value change in update interval and sends data to Message Handling Loop"
        n121 = event-data() -> ("NewVal"=w411:u32)  [unwired: 1 in]
        n122 = To Variant(anything=w411) -> (Variant=w410:variant)
        n123 = call "Enqueue Message (Single).vi"("Message Data"=w410, "Message"="Update Interval", "Message Queue"=w413) -> ("error out"=w412:errorcluster, "dup Message Queue"=w414:refnum<queue>)  [unwired: 7 in]
      }
      event "Log Events?": Value Change {
        # "Captures value change in Log Events and sends data to Message Handling Loop"
        n124 = event-data() -> ("NewVal"=w416:bool)  [unwired: 1 in]
        n125 = To Variant(anything=w416) -> (Variant=w419:variant)
        n126 = call "Enqueue Message (Single).vi"("Message Data"=w419, "Message"="Update Log Events", "Message Queue"=w418) -> ("dup Message Queue"=w417:refnum<queue>)  [unwired: 7 in, 1 out]
      }
      event "Start": Value Change {
        # "Captures value change in height and enqueues a state for Message Handling Loop"
        n127 = event-data() -> ()  [unwired: 1 in, 1 out]
        n128 = call "Enqueue Message (Single).vi"("Message"="Update Start Game", "Message Queue"=w422) -> ("error out"=w421:errorcluster, "dup Message Queue"=w423:refnum<queue>)  [unwired: 8 in]
      }
      event Panel Close? {
        # "Send the 'Confirm Quit' message if the user closes the panel of the VI. Discard the event so the 'Confirm Quit' message has a chance to run."
        n129 = event-data() -> ()  [unwired: 1 in, 1 out]
        n130 = call-poly "Enqueue Message.vi"("Priority Message? (F)"=TRUE, "Message"="Confirm Quit", "Message Queue"=w429) -> ("error out"=w428:errorcluster, "dup Message Queue"=w427:refnum<queue>)  [unwired: 7 in]
        n131 = event-data("Discard?"=TRUE) -> ()  [unwired: 1 in, 1 out]
      }
      event Application Instance Close {
        # "#CodeRecommended - When a project closes, all VIs within that project are aborted and leave memory. However, any code placed in this event frame is guaranteed to run to completion, so add any cleanup code that absolutely must happen here."
        n132 = event-data() -> ()  [unwired: 1 in, 1 out]
      }
      event User Event {
        # "The Message Handling Loop processed an \"Exit\" message, which fired this event to stop the Event Handling Loop."
        n133 = event-data() -> ()  [unwired: 1 in, 1 out]
      }
    }
    n134 = call "Error Handler - Event Handling Loop.vi"("error in (no error)"=w374, "Message Queue"=w372) -> ("dup error in"=w371:errorcluster)  [unwired: 8 in, 1 out]
  }
  n135 = Unregister For Events(event registration refnum=w19, error in=w18) -> (error out=w20:errorcluster)
  n136 = Merge Errors(w20, w24) -> (w21:errorcluster)
  n137 = call "Destroy User Event - Stop.vi"("error in (no error)"=w21, "User Event - Stop"=w17) -> ("error out"=w5:errorcluster)  [unwired: 9 in]
  n138 = call <vilib>:"Close Session.vi"("error in (no error)"=w5, "Session in"=w6) -> ("error out"=w4:errorcluster)  [unwired: 9 in]
  n139 = disable-structure shown="RUN_TIME_ENGINE==True" {
    disable-tunnel: w4 -> [_ _]
    frame condition #0 (active) {
    }
    frame condition #1 {
      # "Call Quit LabVIEW if running as a built application."
      n140 = Quit LabVIEW() -> ()  [unwired: 1 in]
    }
  }
